vi "Measurement UI.vi"() -> ()   [LabVIEW 2025, in "Fgen Script Mode UI.lvlib"]
uses:
  Fgen Script Mode UI.lvlib
  Typedef/Script Meas Config Ctrl Ref.ctl
  Typedef/Script UI Ctrl Ref.ctl
  Typedef/Waveforms UI Ctrl Ref.ctl
  Typedef/Waveform Meas Config Ctrl Ref.ctl
  <vilib>/Platform/browser.llb/Open URL in Default Browser (string).vi
panel:
  out "Actual Sample Rate":dbl format="%#_6pHz"
  in  "Go to Script Help":bool
  out "Waveform Preview":waveform(dbl)(graph)
  in  "Change Waveform":bool
  in  "Trigger Settings":bool
  in  "Remove Selected Waveform":bool
  in  "Add Waveform":bool
  in  "Selected Waveform":u16(ring) items=["Wfm0"]
  in  "Script Body":string
  out "Script Footer":string="Script End"
  out "Script Header":string="Script"
  in  "Script Names":string[](array[string])
  in  "Remove Selected Script":bool
  in  "Add Script":bool
  in  "Selected Script (Ring)":u16(ring) caption="Selected Script"
  in  "Selected Script":string
  in  "Script Trigger Settings":string
  in  "Waveforms":string[](array[string])
  in  "Scripts":string[](array[string])
  in  "FGEN Resource Name":string(combo)
  # "Script"
  # "Waveform"
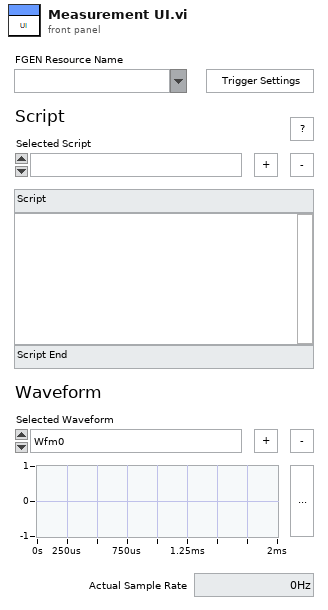
[diagram p1: front panel]
types:
  T1 = typedef "Fgen Script Mode UI.lvlib/Waveform Meas Config Ctrl Ref.ctl" = cluster{"Waveforms Ref":refnum<vi>}
  T2 = typedef "Fgen Script Mode UI.lvlib/Waveforms UI Ctrl Ref.ctl" = cluster{"Selected Waveform Ref (Ring)":refnum<vi>, "Waveform Preview":refnum<vi>, "Change Waveform Ref":refnum<vi>}
  T3 = typedef "Fgen Script Mode UI.lvlib/Script UI Ctrl Ref.ctl" = cluster{"Script Body Ref":refnum<vi>, "Selected Script (Ring) Ref":refnum<vi>, "Script Header Ref":refnum<vi>}
  T4 = typedef "Fgen Script Mode UI.lvlib/Script Meas Config Ctrl Ref.ctl" = cluster{"Scripts Ref":refnum<vi>, "Script Names Ref":refnum<vi>, "Selected Script":refnum<vi>}
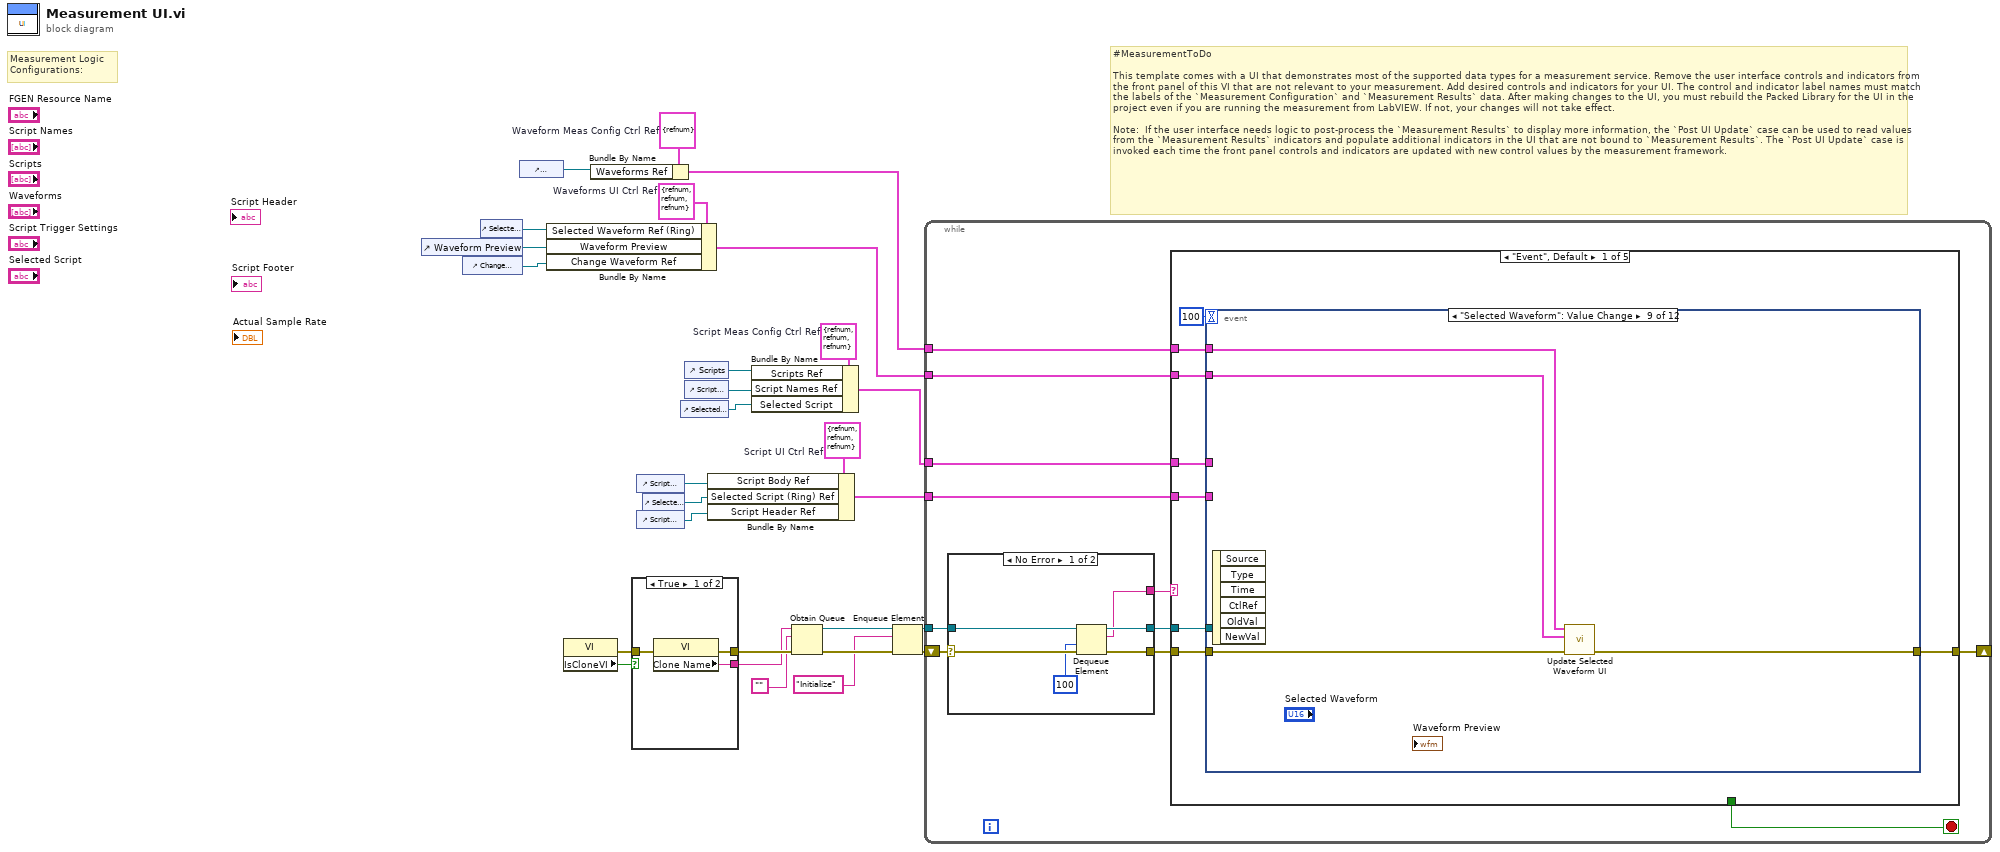
[diagram p0: block diagram]
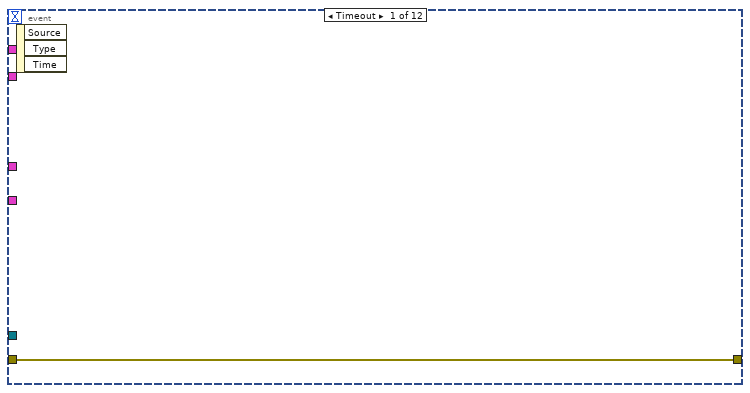
[diagram p2: hidden frame]
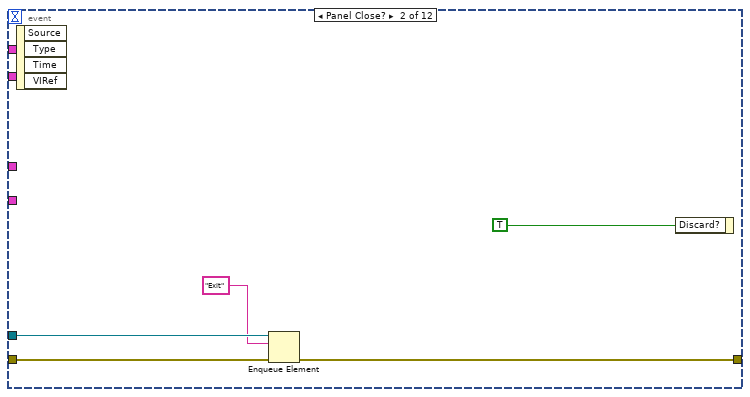
[diagram p3: hidden frame]
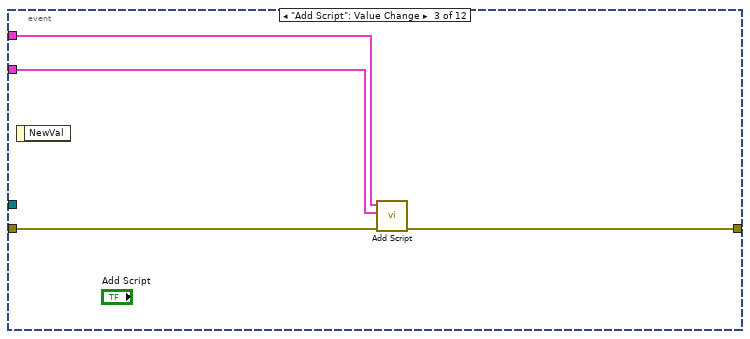
[diagram p4: hidden frame]
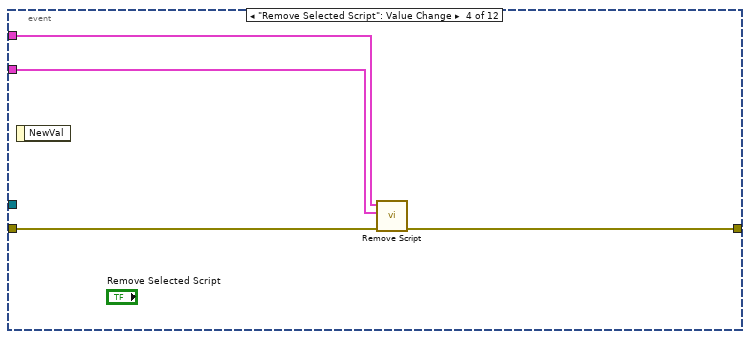
[diagram p5: hidden frame]
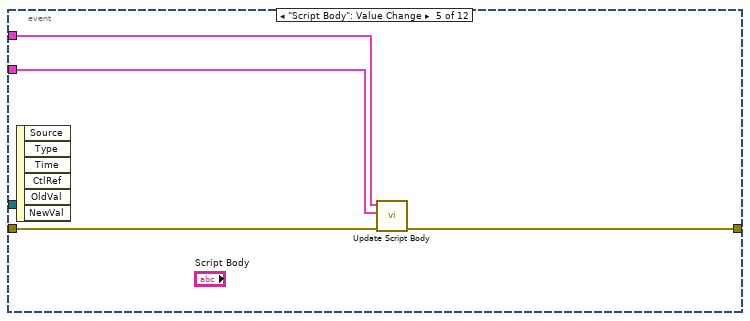
[diagram p6: hidden frame]
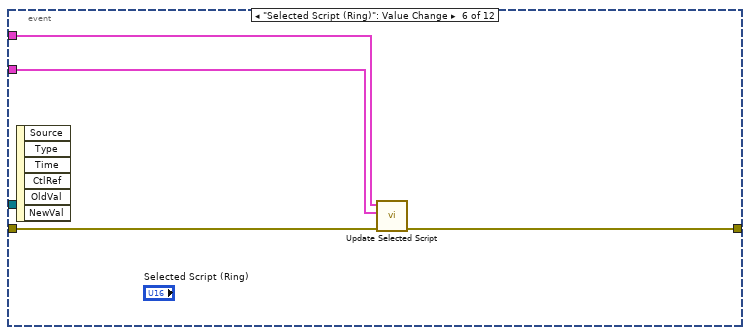
[diagram p7: hidden frame]
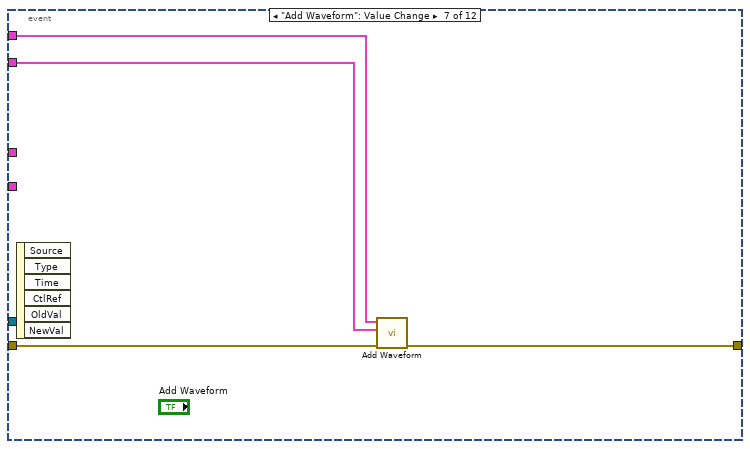
[diagram p8: hidden frame]
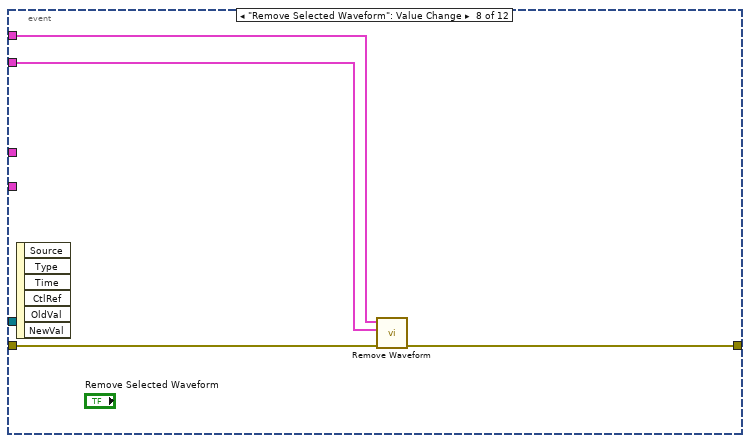
[diagram p9: hidden frame]
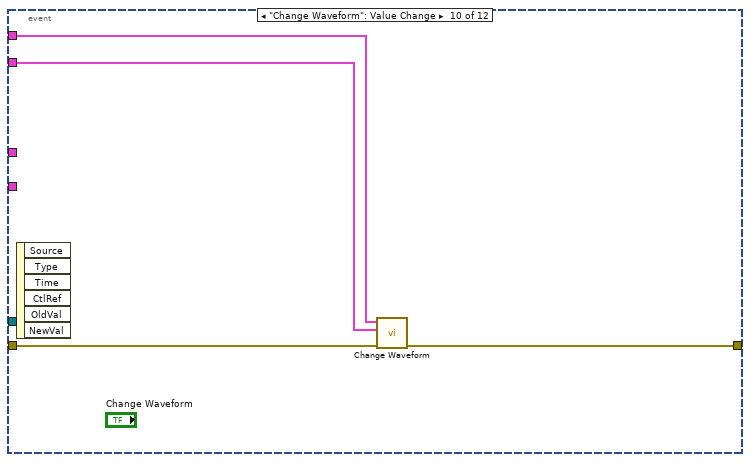
[diagram p10: hidden frame]
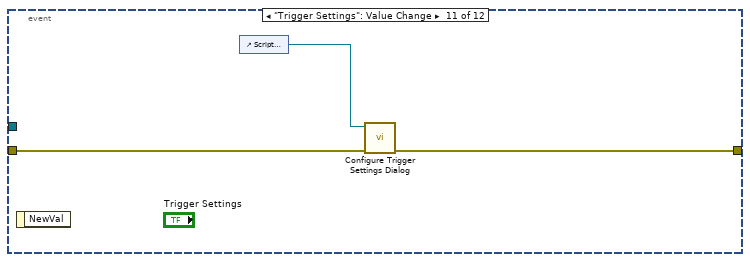
[diagram p11: hidden frame]
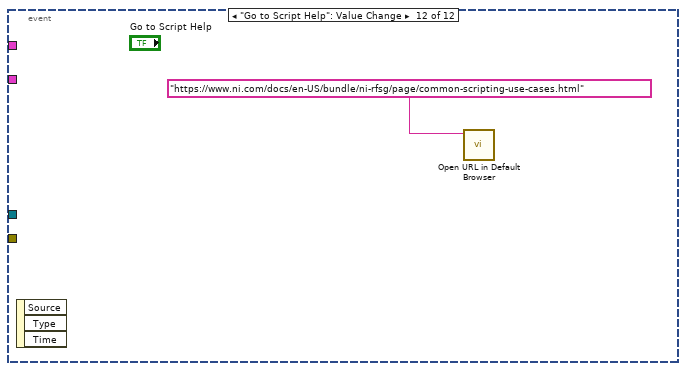
[diagram p12: hidden frame]
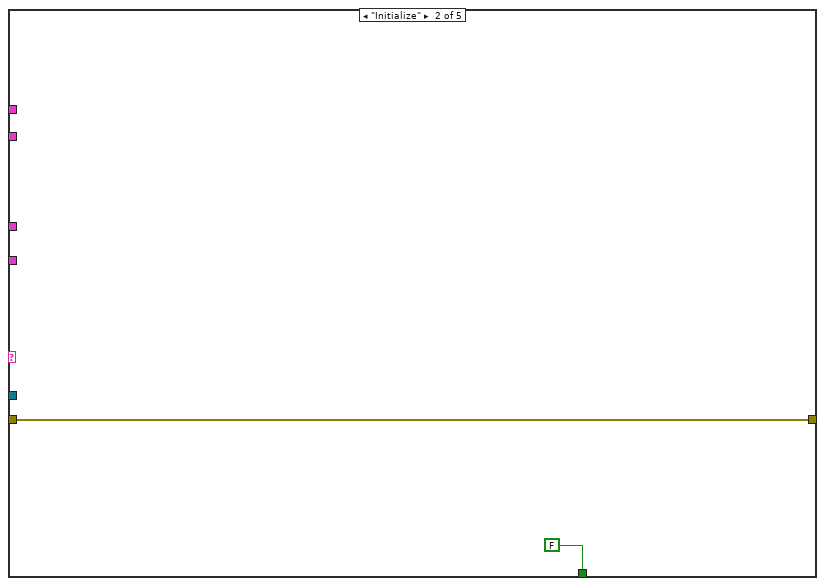
[diagram p13: hidden frame]
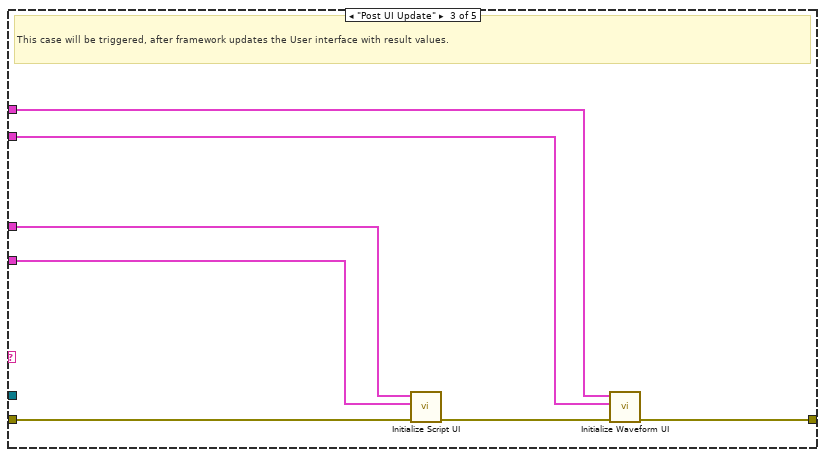
[diagram p14: hidden frame]
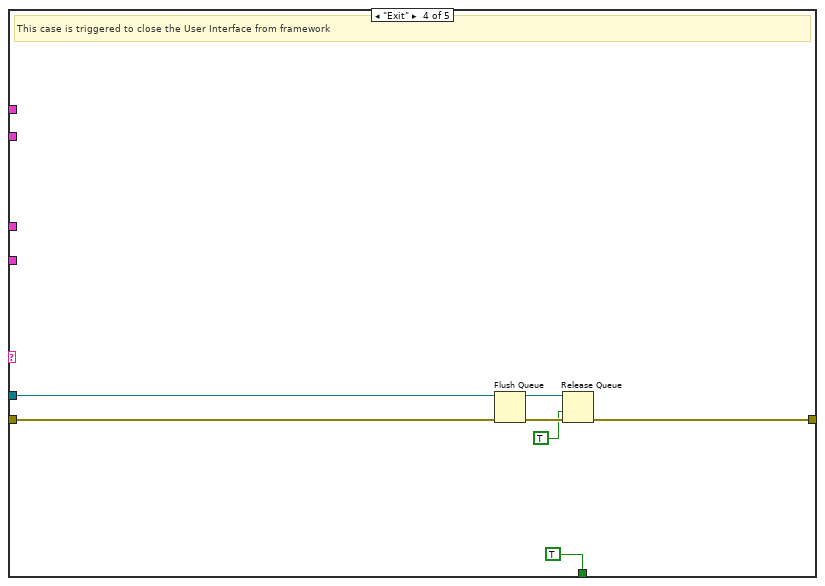
[diagram p15: hidden frame]
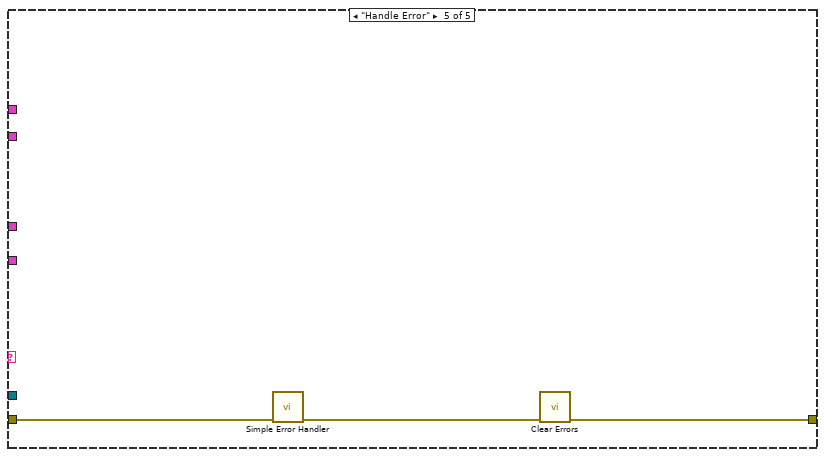
[diagram p16: hidden frame]
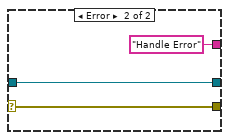
[diagram p17: hidden frame]
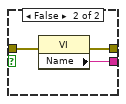
[diagram p18: hidden frame]
diagram:
  w7 = T1 {"Waveforms Ref"=refnum}  # Waveform Meas Config Ctrl Ref
  w5 = T2 {"Selected Waveform Ref (Ring)"=refnum, "Waveform Preview"=refnum, "Change Waveform Ref"=refnum}  # Waveforms UI Ctrl Ref
  w17 = T3 {"Script Body Ref"=refnum, "Selected Script (Ring) Ref"=refnum, "Script Header Ref"=refnum}  # Script UI Ctrl Ref
  w18 = T4 {"Scripts Ref"=refnum, "Script Names Ref"=refnum, "Selected Script"=refnum}  # Script Meas Config Ctrl Ref
  # "Measurement Logic \nConfigurations:"
  # "#MeasurementToDo  \n\nThis template comes with a UI that demonstrates most of the supported data types for a measurement service. Remove the user interface controls and indicators from the front panel of this VI that are not relevant to your measurement. Add desired controls and indicators for your UI. The control and indicator label names must match the labels of the `Measurement Configuration` and `Measurement Results` data. After making changes to the UI, you must rebuild the Packed Library for the UI in the project even if you are running the measurement from LabVIEW. If not, your changes will not take effect.\n\nNote:  If the user interface needs logic to post-process the `Measurement Results` to display more information, the `Post UI Update` case can be used to read values from the `Measurement Results` indicators and populate additional indicators in the UI that are not bound to `Measurement Results`. The `Post UI Update` case is invoked each time the front panel controls and indicators are updated with new control values by the measurement framework."
  n1 = control-ref of="Waveform Preview"() -> (w2:refnum<vi>)
  n2 = control-ref of="Change Waveform"() -> (w1:refnum<vi>)
  n3 = control-ref of="Selected Waveform"() -> (w6:refnum<vi>)
  n4 = control-ref of="Waveforms"() -> (w8:refnum<vi>)
  n5 = Bundle By Name(cluster=w5, "Selected Waveform Ref (Ring)"=w6, "Waveform Preview"=w2, "Change Waveform Ref"=w1) -> (w4:T2)
  n6 = property class="VI"() -> (error out=w19:errorcluster, "IsCloneVI"=w20:bool)  [unwired: 2 in, 1 out]
  n7 = Bundle By Name(cluster=w7, "Waveforms Ref"=w8) -> (w3:T1)
  n8 = case shown="True" w20 {
    tunnel: [w31 w34] -> w28
    tunnel: [w30 w33] -> w27
    tunnel: w19 -> [w29 w32]
    frame True {
      n9 = property class="VI"(error in=w29) -> (error out=w31:errorcluster, "Clone Name"=w30:string)  [unwired: 1 in, 1 out]
    }
    frame False {
      n10 = property class="VI"(error in=w32) -> (error out=w34:errorcluster, "Name"=w33:string)  [unwired: 1 in, 1 out]
    }
  }
  n11 = control-ref of="Script Body"() -> (w11:refnum<vi>)
  n12 = control-ref of="Script Header"() -> (w9:refnum<vi>)
  n13 = control-ref of="Selected Script (Ring)"() -> (w10:refnum<vi>)
  n14 = control-ref of="Selected Script"() -> (w13:refnum<vi>)
  n15 = control-ref of="Scripts"() -> (w15:refnum<vi>)
  n16 = control-ref of="Script Names"() -> (w14:refnum<vi>)
  n17 = Bundle By Name(cluster=w17, "Script Body Ref"=w11, "Selected Script (Ring) Ref"=w10, "Script Header Ref"=w9) -> (w12:T3)
  n18 = Bundle By Name(cluster=w18, "Scripts Ref"=w15, "Script Names Ref"=w14, "Selected Script"=w13) -> (w16:T4)
  n19 = Obtain Queue(name (unnamed)=w27, element data type="", error in (no error)=w28) -> (queue out=w24:refnum<queue>, error out=w26:errorcluster)  [unwired: 2 in, 1 out]
  n20 = Enqueue Element(queue=w24, element="Initialize", error in (no error)=w26) -> (queue out=w23:refnum<queue>, error out=w25:errorcluster)  [unwired: 1 in, 1 out]
  n21 = while {
    shift-right: [w40] -> _
    shift-left: w25 -> [w45]
    tunnel: w23 -> [w43]
    tunnel: w16 -> [w38]
    tunnel: w12 -> [w37]
    tunnel: w4 -> [w36]
    tunnel: w3 -> [w35]
    stop <- w39 stop-if-true
    n22 = case shown="No Error" w45 {
      selector: w45 -> [w120 w123]
      tunnel: [w119 w123] -> w44
      tunnel: w43 -> [w118 w122]
      tunnel: [w117 w122] -> w42
      tunnel: [w116 "Handle Error"] -> w41
      frame No Error {
        n23 = Dequeue Element(queue=w118, timeout in ms (-1)=100, error in (no error)=w120) -> (queue out=w117:refnum<queue>, element=w116:string, error out=w119:errorcluster)  [unwired: 1 out]
      }
      frame Error {
      }
    }
    n24 = case shown="\"Event\", Default" w41 {
      tunnel: w44 -> [w52 w97 w104 w111 w114]
      tunnel: w42 -> [w50 _ _ w109 _]
      tunnel: [w53 w97 w100 w106 w112] -> w40
      tunnel: [_ FALSE _ TRUE _] -> w39
      tunnel: w38 -> [w49 _ w102 _ _]
      tunnel: w37 -> [w48 _ w101 _ _]
      tunnel: w36 -> [w46 _ w98 _ _]
      tunnel: w35 -> [w47 _ w99 _ _]
      frame "Event", Default {
        n25 = event shown="[8] \"Selected Waveform\": Value Change" {
          selector: _ -> [_ _ _ _ _ _ _ _ _ _ _ _]
          dyn-events: _ -> [_ _ _ _ _ _ _ _ _ _ _ _]
          timeout: 100 -> [_ _ _ _ _ _ _ _ _ _ _ _]
          tunnel: [w54 w57 w62 w66 w70 w74 w78 w82 w86 w90 w93 _] -> w53
          tunnel: w52 -> [w54 w58 w63 w67 w71 w75 w79 w83 w87 w91 w94 _]
          tunnel: w50 -> [_ w56 _ _ _ _ _ _ _ _ _ _]
          tunnel: w49 -> [_ _ w61 w65 w69 w73 _ _ _ _ _ _]
          tunnel: w48 -> [_ _ w60 w64 w68 w72 _ _ _ _ _ _]
          tunnel: w47 -> [_ _ _ _ _ _ w77 w81 w85 w89 _ _]
          tunnel: w46 -> [_ _ _ _ _ _ w76 w80 w84 w88 _ _]
          event Timeout {
            n26 = event-data() -> ()  [unwired: 1 in, 3 out]
          }
          event Panel Close? {
            n27 = event-data() -> ()  [unwired: 1 in, 4 out]
            n28 = Enqueue Element(queue=w56, element="Exit", error in (no error)=w58) -> (error out=w57:errorcluster)  [unwired: 1 in, 2 out]
            n29 = event-data("Discard?"=TRUE) -> ()  [unwired: 1 in, 1 out]
          }
          event "Add Script": Value Change {
            n30 = event-data() -> ()  [unwired: 1 in, 1 out]
            n31 = call "Add Script.vi"("error in"=w63, "Script UI Ctrl Ref"=w60, "Script Meas Config Ctrl Ref"=w61) -> ("error out"=w62:errorcluster)  [unwired: 8 in]
          }
          event "Remove Selected Script": Value Change {
            n32 = event-data() -> ()  [unwired: 1 in, 1 out]
            n33 = call "Remove Script.vi"("error in"=w67, "Script UI Ctrl Ref"=w64, "Script Meas Config Ctrl Ref"=w65) -> ("error out"=w66:errorcluster)  [unwired: 8 in]
          }
          event "Script Body": Value Change {
            n34 = event-data() -> ()  [unwired: 1 in, 6 out]
            n35 = call "Update Script Body.vi"("error in"=w71, "Script UI Ctrl Ref"=w68, "Script Meas Config Ctrl Ref"=w69) -> ("error out"=w70:errorcluster)  [unwired: 8 in]
          }
          event "Selected Script (Ring)": Value Change {
            n36 = event-data() -> ()  [unwired: 1 in, 6 out]
            n37 = call "Update Selected Script.vi"("error in"=w75, "Script UI Ctrl Ref"=w72, "Script Meas Config Ctrl Ref"=w73) -> ("error out"=w74:errorcluster)  [unwired: 8 in]
          }
          event "Add Waveform": Value Change {
            n38 = event-data() -> ()  [unwired: 1 in, 6 out]
            n39 = call "Add Waveform.vi"("error in"=w79, "Waveforms UI Ctrl Ref"=w76, "Waveform Meas Config Ctrl Ref"=w77) -> ("error out"=w78:errorcluster)  [unwired: 8 in]
          }
          event "Remove Selected Waveform": Value Change {
            n40 = event-data() -> ()  [unwired: 1 in, 6 out]
            n41 = call "Remove Waveform.vi"("error in"=w83, "Waveforms UI Ctrl Ref"=w80, "Waveform Meas Config Ctrl Ref"=w81) -> ("error out"=w82:errorcluster)  [unwired: 8 in]
          }
          event "Selected Waveform": Value Change {
            n42 = event-data() -> ()  [unwired: 1 in, 6 out]
            n43 = call "Update Selected Waveform UI.vi"("error in"=w87, "Waveforms UI Ctrl Ref"=w84, "Waveform Meas Config Ctrl Ref"=w85) -> ("error out"=w86:errorcluster)  [unwired: 8 in]
          }
          event "Change Waveform": Value Change {
            n44 = event-data() -> ()  [unwired: 1 in, 6 out]
            n45 = call "Change Waveform.vi"("error in"=w91, "Waveforms UI Ctrl Ref"=w88, "Waveform Meas Config Ctrl Ref"=w89) -> ("error out"=w90:errorcluster)  [unwired: 8 in]
          }
          event "Trigger Settings": Value Change {
            n46 = event-data() -> ()  [unwired: 1 in, 1 out]
            n47 = control-ref of="Script Trigger Settings"() -> (w92:refnum<vi>)
            n48 = call "Configure Trigger Settings Dialog.vi"("error in"=w94, "Script Trigger Settings Ref"=w92) -> ("error out"=w93:errorcluster)  [unwired: 9 in]
          }
          event "Go to Script Help": Value Change {
            n49 = event-data() -> ()  [unwired: 1 in, 3 out]
            n50 = call-poly <vilib>:"Open URL in Default Browser.vi"("URL"="https://www.ni.com/docs/en-US/bundle/ni-rfsg/page/common-scripting-use-cases.html") -> ()  [unwired: 5 in, 2 out]
          }
        }
      }
      frame "Initialize" {
      }
      frame "Post UI Update" {
        # "This case will be triggered, after framework updates the User interface with result values."
        n51 = call "Initialize Script UI.vi"("error in"=w104, "Script UI Ctrl Ref"=w101, "Script Meas Config Ctrl Ref"=w102) -> ("error out"=w103:errorcluster)  [unwired: 8 in]
        n52 = call "Initialize Waveform UI.vi"("error in"=w103, "Waveforms UI Ctrl Ref"=w98, "Waveform Meas Config Ctrl Ref"=w99) -> ("error out"=w100:errorcluster)  [unwired: 8 in]
      }
      frame "Exit" {
        # "This case is triggered to close the User Interface from framework"
        n53 = Flush Queue(queue=w109, error in (no error)=w111) -> (queue out=w108:refnum<queue>, error out=w107:errorcluster)  [unwired: 1 out]
        n54 = Release Queue(queue=w108, force destroy? (F)=TRUE, error in (no error)=w107) -> (error out=w106:errorcluster)  [unwired: 2 out]
      }
      frame "Handle Error" {
        n55 = call <vilib>:"Simple Error Handler.vi"("error in (no error)"=w114) -> ("error out"=w113:errorcluster)  [unwired: 4 in, 4 out]
        n56 = call <vilib>:"Clear Errors.vi"("error in (no error)"=w113) -> ("error out"=w112:errorcluster)  [unwired: 5 in, 1 out]
      }
    }
  }
